vi "Read Test Case Result.vi"(11 "LUnit Test Case In":refnum<class "LUnit Test Case.lvclass">) -> (2 "Test Case Result":T1, 3 "LUnit Test Case Out":refnum<class "LUnit Test Case.lvclass">)   [LabVIEW 2020, in "LUnit Test Case.lvclass"]
uses:
  LUnit Test Case.lvclass
  Result Types/Assertion Result/Public/TypeDefs/Status.ctl
  Result Types/Assertion Result/Assertion Result.lvlib
  Result Types/Assertion Result/Public/TypeDefs/Assertion Type.ctl
  Result Types/Assertion Result/Assertion Result.ctl
  Result Types/Method Result/Method Result.ctl
  Result Types/Method Result/Method Result.lvlib
  Result Types/Case Result/Test Case Result.ctl
  Result Types/Case Result/Test Case Result.lvlib
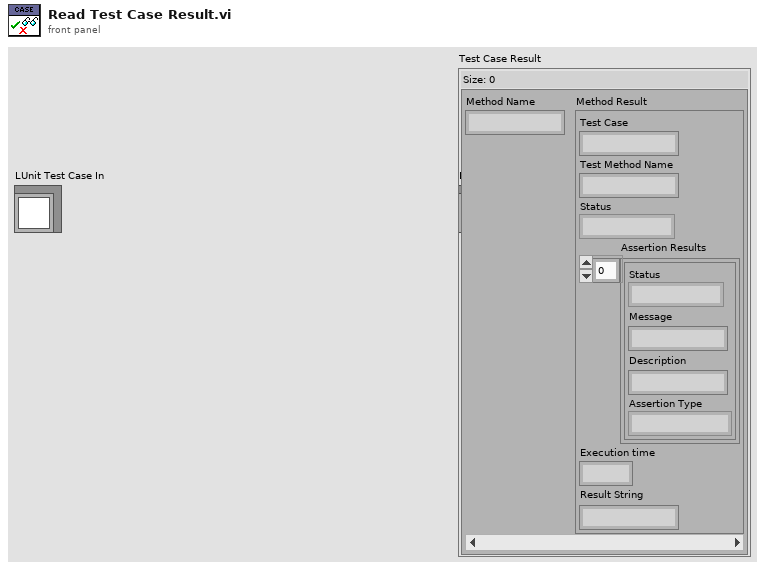
[diagram p1: front panel]
types:
  T1 = typedef "Test Case Result.lvlib/Test Case Result.ctl" = map{string, T2}
  T2 = typedef "Method Result.lvlib/Method Result.ctl" = cluster{"Test Case":string, "Test Method Name":string, "Status":T3, "Assertion Results":T4[], "Execution time":dbl, "Result String":string}
  T3 = typedef "Assertion Result.lvlib/Status.ctl" = enum16{"Pass", "Fail", "Error", "Skipped", "Setup Error", "Broken", "Teardown Error"}
  T4 = typedef "Assertion Result.lvlib/Assertion Result.ctl" = cluster{"Status":T3, "Message":string, "Description":string, "Assertion Type":T5}
  T5 = typedef "Assertion Result.lvlib/Assertion Type.ctl" = enum16{"None", "Pass", "Fail", "Skip", "Pass if Equal", "Fail if Equal", "Pass if Error", "Fail if Error", "Pass if", "Fail if"}
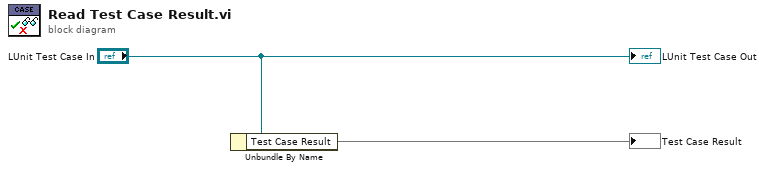
[diagram p0: block diagram]
diagram:
  n1 = Unbundle By Name("LUnit Test Case In") -> ("Test Case Result"=→"Test Case Result":T1)
  "LUnit Test Case Out" <- "LUnit Test Case In"
